vi "Online_Program_redesign_For_TV.vi"() -> ()   [LabVIEW 2014]
uses:
  <vilib>/Utility/file.llb/Read From Spreadsheet File (DBL).vi
  <vilib>/Analysis/Matrix/Numeric/Conversions/Array To Matrix - RA2.vi
  <vilib>/Instr/_visa.llb/VISA Configure Serial Port (Instr).vi
  <vilib>/Analysis/Matrix/Numeric/Conversions/Array To Matrix - RA.vi
  <vilib>/Utility/file.llb/Write To Spreadsheet File (DBL).vi
  <vilib>/Utility/file.llb/Write To Spreadsheet File (I64).vi
  <vilib>/Analysis/Matrix/NI_Matrix.lvlib
  NeuroSky_Dll_Call/Debug/NeuroSky_Dll_Call.dll
  user32.dll
panel:
  out "에러 출력":errorcluster
  out "메시지 2":string
  out "큐사인":bool
  out "icon_온도":bool
  out "icon_용변":bool
  out "icon_자판":bool
  out "icon_응급":bool=TRUE
  out "icon_기계":bool
  out "icon_침대":bool
  out "메시지":string
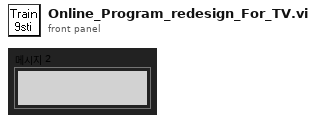
[diagram p1: front panel]
types:
  T1 = typedef "NI_Matrix.lvlib/RealMatrix.ctl" = dbl[][]
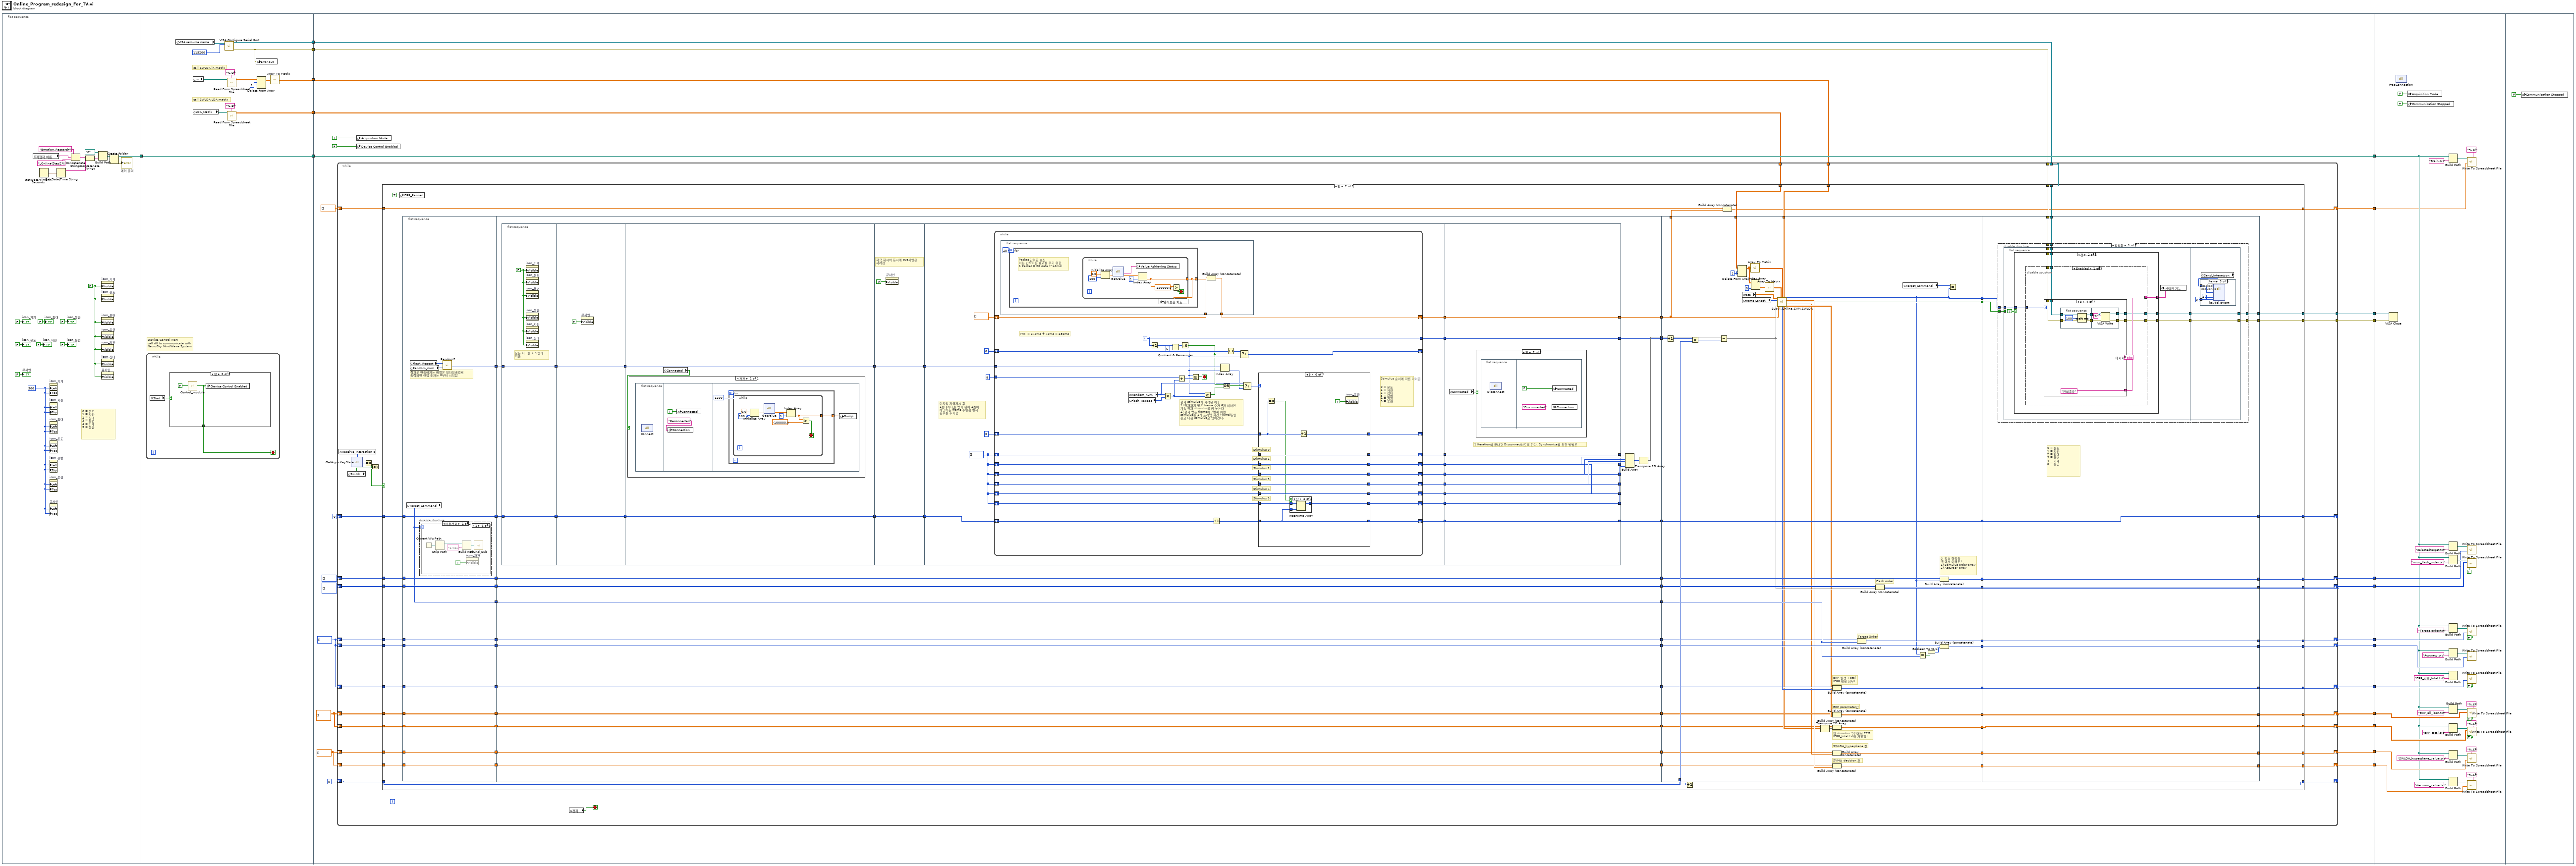
[diagram p0: block diagram]
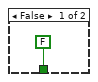
[diagram p2: hidden frame]
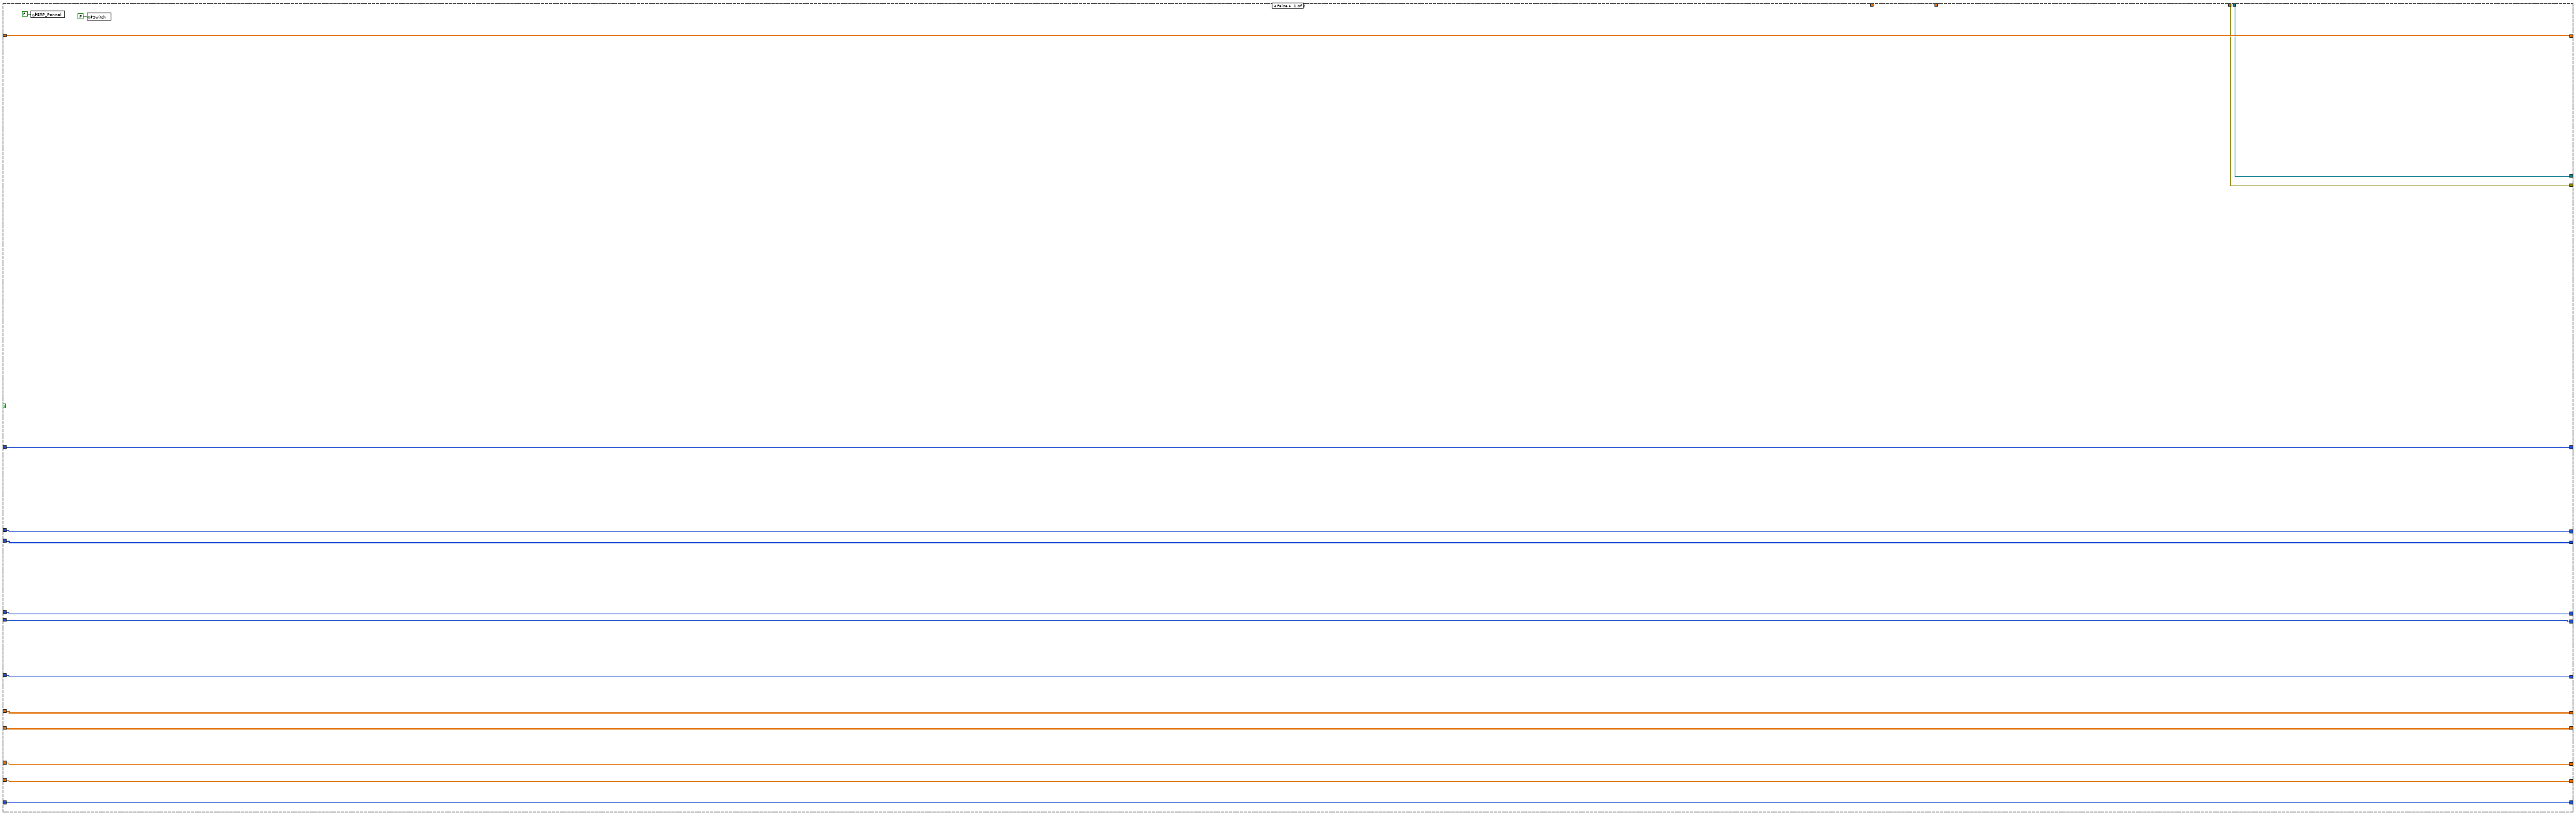
[diagram p3: hidden frame]
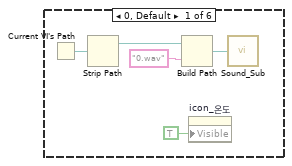
[diagram p4: hidden frame]
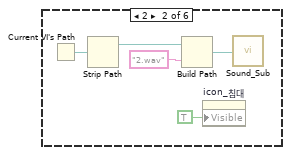
[diagram p5: hidden frame]
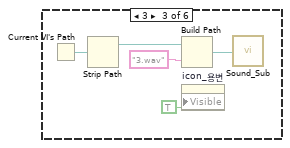
[diagram p6: hidden frame]
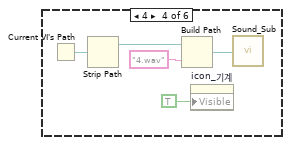
[diagram p7: hidden frame]
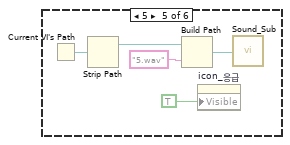
[diagram p8: hidden frame]
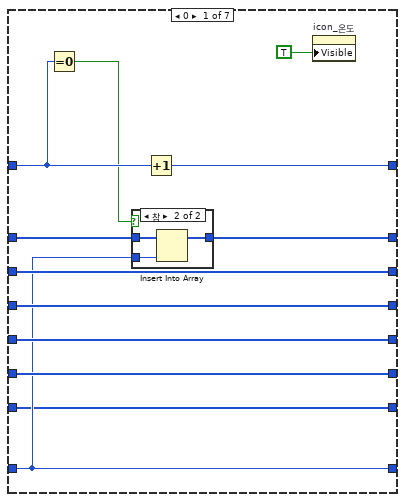
[diagram p11: hidden frame]
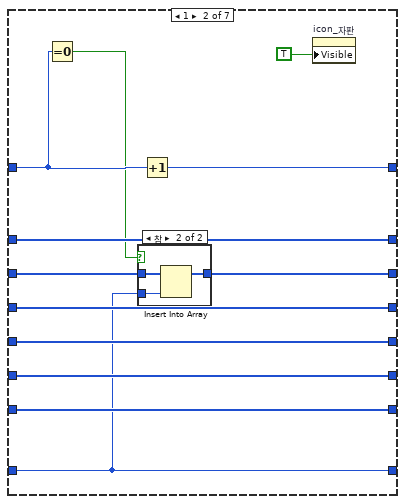
[diagram p13: hidden frame]
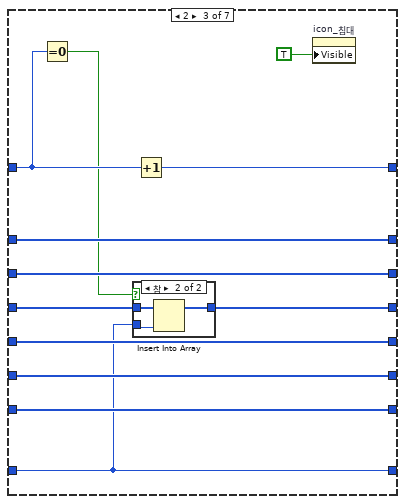
[diagram p15: hidden frame]
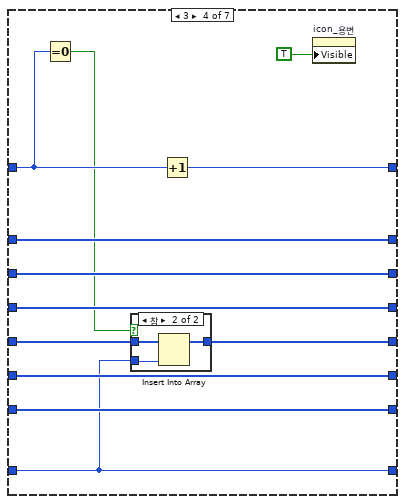
[diagram p17: hidden frame]
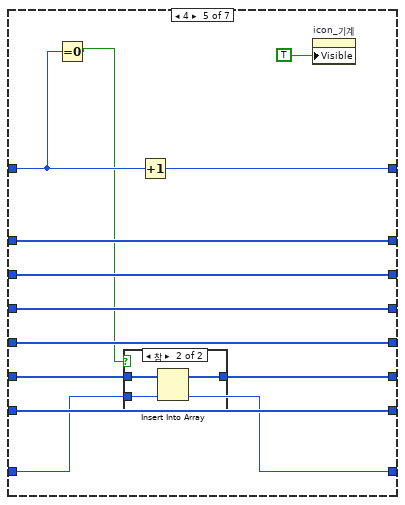
[diagram p19: hidden frame]
diagram:
  n1 = flat-sequence {
    tunnel: [w39] -> w19
    tunnel: w19 -> [w53]
    tunnel: [w53] -> w18
    tunnel: [w51] -> w17
    tunnel: [w44] -> w7
    tunnel: [w43] -> w4
    tunnel: [w40] -> w3
    tunnel: w18 -> [w76]
    tunnel: [w76] -> w16
    tunnel: [w85] -> w15
    tunnel: [w83] -> w14
    tunnel: [w81] -> w13
    tunnel: w17 -> [w65]
    tunnel: [w80] -> w12
    tunnel: [w77] -> w11
    tunnel: [w73] -> w10
    tunnel: [w71] -> w9
    tunnel: [w70] -> w8
    tunnel: w7 -> [w64]
    tunnel: [w68] -> w6
    tunnel: [w66] -> w5
    tunnel: w4 -> [w63]
    tunnel: w3 -> [w62]
    tunnel: [w61] -> w2
    tunnel: [w60] -> w1
    tunnel: w16 -> [w774]
    tunnel: w15 -> [w769]
    tunnel: w14 -> [w808]
    tunnel: w13 -> [w804]
    tunnel: w12 -> [w801]
    tunnel: w11 -> [w797]
    tunnel: w10 -> [w791]
    tunnel: w9 -> [w786]
    tunnel: w8 -> [w783]
    tunnel: w6 -> [w780]
    tunnel: w5 -> [w775]
    tunnel: w2 -> [w771]
    tunnel: w1 -> [w770]
    frame #0 {
      w20 = FALSE ("Visible")
      w22 = 500 ("Position:Left")
      # "0 = 온도\n1 = 자판\n2 = 침대\n3 = 용변 \n4 = 기계 \n5 = 응급"
      n2 = global read "Control_Panel_정리.vi" "피험자 이름"() -> (w30:string)
      n3 = Get Date/Time In Seconds() -> (seconds since 1Jan1904=w36:timestamp)
      n4 = property on="icon_기계" class="Bool (엄격한)"("Left"=w22, "Top"=w22) -> ()  [unwired: 2 in, 2 out]
      n5 = property on="icon_자판" class="Bool (엄격한)"("Left"=w22, "Top"=w22) -> ()  [unwired: 2 in, 2 out]
      n6 = property on="icon_침대" class="Bool (엄격한)"("Left"=w22, "Top"=w22) -> ()  [unwired: 2 in, 2 out]
      n7 = property on="icon_온도" class="Bool (엄격한)"("Left"=w22, "Top"=w22) -> ()  [unwired: 2 in, 2 out]
      n8 = property on="icon_용변" class="Bool (엄격한)"("Left"=w22, "Top"=w22) -> ()  [unwired: 2 in, 2 out]
      n9 = property on="icon_응급" class="Bool (엄격한)"("Left"=w22, "Top"=w22) -> ()  [unwired: 2 in, 2 out]
      n10 = property on="큐사인" class="Bool (엄격한)"("Left"=w22, "Top"=w22) -> ()  [unwired: 2 in, 2 out]
      n11 = Get Date/Time String(seconds (now)=w36) -> (date string=w37:string)  [unwired: 2 in, 1 out]
      n12 = Concatenate Strings("Emotion_Research\\" ("string"), w30, "_Online(Step2)\\" ("문자열")) -> (w32:string)
      n13 = Concatenate Strings(w32, w37) -> (w34:string)
      n14 = Build Path(base path=path "C:/" ("path"), name or relative path=w34) -> (appended path=w35:path)
      n15 = property on="icon_기계" class="Bool (엄격한)"("Visible"=w20) -> ()  [unwired: 2 in, 2 out]
      n16 = property on="icon_온도" class="Bool (엄격한)"("Visible"=w20) -> ()  [unwired: 2 in, 2 out]
      n17 = property on="icon_용변" class="Bool (엄격한)"("Visible"=w20) -> ()  [unwired: 2 in, 2 out]
      n18 = property on="icon_응급" class="Bool (엄격한)"("Visible"=w20) -> ()  [unwired: 2 in, 2 out]
      n19 = property on="icon_자판" class="Bool (엄격한)"("Visible"=w20) -> ()  [unwired: 2 in, 2 out]
      n20 = property on="icon_침대" class="Bool (엄격한)"("Visible"=w20) -> ()  [unwired: 2 in, 2 out]
      n21 = property on="큐사인" class="Bool (엄격한)"("Visible"=w20) -> ()  [unwired: 2 in, 2 out]
      n22 = Create Folder(path (use dialog)=w35) -> (created path=w39:path, error out=→"에러 출력":errorcluster)  [unwired: 2 in, 1 out]
      "icon_온도" <- FALSE ("icon_전원 6")
      "icon_용변" <- FALSE ("icon_전체종료")
      "icon_자판" <- FALSE ("icon_음량업 2")
      "icon_응급" <- FALSE ("icon_채널다운")
      "icon_기계" <- FALSE ("icon_음량다")
      "icon_침대" <- FALSE ("icon_채널업")
      "큐사인" <- FALSE ("icon_전원 7")
    }
    frame #1 {
      w47 = 1 ("인덱스 (행)")
      # "call SWLDA in matrix"
      # "call SWLDA LDA matrix"
      # "Device Control Part\ncall dll to communicate with\nNeuroSky MindWave System"
      n23 = while {
        stop <- w55 stop-if-true
        n24 = global read "Control_Panel_정리.vi" "Start"() -> (w54:bool)
        n25 = case shown="참" w54 {
          tunnel: [FALSE ("Connected") w57] -> w55
          frame False {
          }
          frame True {
            n26 = call "Control_module.vi"("Turn on"=TRUE ("Device Control Enabled")) -> ("Connected"=w57:bool)
            n27 = global write "Control_Panel_정리.vi" "Device Control Enabled"(w57) -> ()
          }
        }
      }
      n28 = global read "Control_Panel_정리.vi" "VISA resource name"() -> (w41:refnum<visa-resource-name>)
      n29 = global read "Control_Panel_정리.vi" "in"() -> (w45:path)
      n30 = global read "Control_Panel_정리.vi" "LDA_Matrix"() -> (w50:path)
      n31 = call-poly "VISA Configure Serial Port"("VISA resource name"=w41, "baud rate (9600)"=u32 115200) -> ("VISA resource name out"=w43:refnum<visa-resource-name>, "error out"=w40:errorcluster)  [unwired: 12 in]
      n32 = call-poly <vilib>:"Read From Spreadsheet File.vi"("format (%.3f)"="%.6f", "file path (dialog if empty)"=w45) -> ("all rows"=w46:dbl[][])  [unwired: 5 in, 4 out]
      n33 = call-poly <vilib>:"Read From Spreadsheet File.vi"("format (%.3f)"="%.6f", "file path (dialog if empty)"=w50) -> ("all rows"=w51:dbl[][])  [unwired: 5 in, 4 out]
      n34 = global write "Control_Panel_정리.vi" "error out"(w40) -> ()
      n35 = Delete From Array(array=w46, length=w47, index (row)=w47) -> (array with subset deleted=w48:dbl[][])  [unwired: 1 in, 1 out]
      n36 = call-poly <vilib>:"Array To Matrix.vi"("Real 2D Array"=w48) -> ("Real Matrix"=w44:T1)
    }
    frame #2 {
      w69 = dbl[] []
      w67 = dbl[][] []
      w72 = i16[] []
      n37 = while {
        shift-right: [w93] -> w85
        shift-left: dbl[] [] -> [w99]
        shift-right: [w119] -> _
        shift-left: 0 ("y") -> [w120]
        shift-right: [w113] -> w83
        shift-left: i32[][] [] -> [w114]
        shift-right: [w117] -> w81
        shift-left: i32[] [] -> [w118]
        shift-right: [w115] -> w80
        shift-left: w72 -> [w116]
        shift-right: [w111] -> w77
        shift-left: w72 -> [w112]
        shift-right: [w110] -> w73
        shift-left: w72 -> [w109]
        shift-right: [w108] -> w71
        shift-left: w67 -> [w107]
        shift-right: [w106] -> w70
        shift-left: w69 -> [w105]
        shift-right: [w104] -> w68
        shift-left: w69 -> [w103]
        shift-right: [w102] -> w66
        shift-left: w67 -> [w101]
        tunnel: w65 -> [w100]
        tunnel: w64 -> [w98]
        tunnel: [w96] -> _
        tunnel: w63 -> [w96]
        tunnel: w62 -> [w97]
        tunnel: [w95] -> w61
        tunnel: [w94] -> w60
        shift-right: [w87] -> _
        shift-left: 0 -> [w88]
        stop <- w89 stop-if-true
        n38 = global read "Control_Panel_정리.vi" "Receive_Interaction"() -> (w91:u8)
        n39 = global read "Control_Panel_정리.vi" "Switch"() -> (w90:bool)
        n40 = dll-call lib="User32.dll" fn="GetAsyncKeyState"("vKey"=w91) -> ("return type"=w92:i64)  [unwired: 4 in, 2 out]
        n41 = Not Equal To 0?(x=w92) -> (x != 0?=w86:bool)
        n42 = Or(x=w86, y=w90) -> ()  [unwired: 1 out]
        n43 = case shown="참" w86 {
          tunnel: w120 -> [w131 w168]
          tunnel: [w131 w167] -> w119
          tunnel: w118 -> [w130 w166]
          tunnel: [w130 w165] -> w117
          tunnel: w116 -> [w127 w164]
          tunnel: [w127 w163] -> w115
          tunnel: w114 -> [w129 w162]
          tunnel: [w129 w161] -> w113
          tunnel: w112 -> [w128 w160]
          tunnel: [w128 w159] -> w111
          tunnel: [w126 w158] -> w110
          tunnel: w109 -> [w126 w157]
          tunnel: [w125 w156] -> w108
          tunnel: w107 -> [w125 w155]
          tunnel: [w123 w154] -> w106
          tunnel: w105 -> [w123 w153]
          tunnel: [w122 w152] -> w104
          tunnel: w103 -> [w122 w151]
          tunnel: [w124 w150] -> w102
          tunnel: w101 -> [w124 w149]
          tunnel: w100 -> [_ w148]
          tunnel: w99 -> [w134 w147]
          tunnel: w98 -> [_ w145]
          tunnel: w97 -> [w132 w144]
          tunnel: w96 -> [w133 w143]
          tunnel: [w133 w142] -> w95
          tunnel: [w132 w141] -> w94
          tunnel: [w134 w140] -> w93
          tunnel: w88 -> [w121 w138]
          tunnel: [w121 w137] -> w87
          frame False {
            n44 = global write "Control_Panel_정리.vi" "ERP_Pannel"(FALSE ("ERP_Pannel")) -> ()
            n45 = global write "Control_Panel_정리.vi" "Switch"(FALSE ("Switch")) -> ()
          }
          frame True {
            n46 = global write "Control_Panel_정리.vi" "ERP_Pannel"(TRUE ("ERP_Pannel")) -> ()
            n47 = flat-sequence {
              tunnel: [w220] -> w206
              tunnel: w168 -> [w219]
              tunnel: [w219] -> w205
              tunnel: [w207] -> w204
              tunnel: w166 -> [w216]
              tunnel: [w216] -> w203
              tunnel: w164 -> [w215]
              tunnel: [w215] -> w202
              tunnel: w162 -> [w214]
              tunnel: [w214] -> w201
              tunnel: [w213] -> w200
              tunnel: w160 -> [w213]
              tunnel: w157 -> [w212]
              tunnel: [w212] -> w199
              tunnel: w155 -> [w211]
              tunnel: [w211] -> w198
              tunnel: w153 -> [w210]
              tunnel: [w210] -> w197
              tunnel: w151 -> [w209]
              tunnel: [w209] -> w196
              tunnel: w149 -> [w208]
              tunnel: [w208] -> w195
              tunnel: w206 -> [w291]
              tunnel: w205 -> [w288]
              tunnel: [w289] -> w194
              tunnel: [w278] -> w193
              tunnel: [w287] -> w192
              tunnel: [w286] -> w191
              tunnel: w204 -> [w285]
              tunnel: [w285] -> w190
              tunnel: w203 -> [w284]
              tunnel: [w284] -> w189
              tunnel: [w283] -> w188
              tunnel: w202 -> [w283]
              tunnel: [w282] -> w187
              tunnel: w201 -> [w282]
              tunnel: [w281] -> w186
              tunnel: w200 -> [w281]
              tunnel: [w280] -> w185
              tunnel: w199 -> [w280]
              tunnel: [w279] -> w184
              tunnel: w198 -> [w279]
              tunnel: [w277] -> w183
              tunnel: w197 -> [w277]
              tunnel: [w276] -> w182
              tunnel: w196 -> [w276]
              tunnel: w195 -> [w275]
              tunnel: [w275] -> w181
              tunnel: w194 -> [w532]
              tunnel: w193 -> [w506]
              tunnel: w192 -> [w545]
              tunnel: w191 -> [w546]
              tunnel: w138 -> [w544]
              tunnel: [w545] -> w170
              tunnel: [w504] -> w171
              tunnel: w190 -> [w531]
              tunnel: w189 -> [w540]
              tunnel: [w539] -> w172
              tunnel: w188 -> [w537]
              tunnel: [w536] -> w173
              tunnel: w187 -> [w535]
              tunnel: [w533] -> w174
              tunnel: w186 -> [w530]
              tunnel: [w529] -> w175
              tunnel: [w527] -> w176
              tunnel: w185 -> [w526]
              tunnel: [w524] -> w177
              tunnel: w184 -> [w523]
              tunnel: [w521] -> w178
              tunnel: w183 -> [w520]
              tunnel: [w518] -> w179
              tunnel: w182 -> [w517]
              tunnel: [w514] -> w180
              tunnel: w181 -> [w513]
              tunnel: w148 -> [w512]
              tunnel: [w506] -> w146
              tunnel: w145 -> [w508]
              tunnel: [w507] -> w169
              tunnel: [w567] -> w167
              tunnel: [w566] -> w165
              tunnel: [w563] -> w163
              tunnel: [w565] -> w161
              tunnel: [w564] -> w159
              tunnel: [w562] -> w158
              tunnel: [w561] -> w156
              tunnel: [w560] -> w154
              tunnel: [w559] -> w152
              tunnel: [w558] -> w150
              tunnel: w180 -> [w558]
              tunnel: w179 -> [w559]
              tunnel: w178 -> [w560]
              tunnel: w177 -> [w561]
              tunnel: w176 -> [w562]
              tunnel: w175 -> [w564]
              tunnel: w174 -> [w565]
              tunnel: w173 -> [w563]
              tunnel: w172 -> [w566]
              tunnel: w171 -> [w557]
              tunnel: w170 -> [w567]
              tunnel: w169 -> [w556]
              tunnel: w144 -> [w555]
              tunnel: w143 -> [w554]
              tunnel: [w553] -> w142
              tunnel: [w552] -> w141
              frame #0 {
                # "결과로 만들어지는 배열은 일차원배열로\n출력되면 랜덤 숫자는 0부터 시작함"
                n48 = global read "Control_Panel_정리.vi" "Target_Command"() -> (w207:i32)
                n49 = global read "Control_Panel_정리.vi" "Flash_Repeat"() -> (w218:i32)
                n50 = global read "Control_Panel_정리.vi" "Random_num"() -> (w217:i32)
                n51 = disable-structure shown="비활성화" {
                  disable-tunnel: w207 -> [w221 _]
                  frame Disabled {
                    n52 = case shown="1" w221 {
                      frame 0, Default {
                        n53 = Current VI's Path() -> (path=w224:path)
                        n54 = Strip Path(path=w224) -> (stripped path=w225:path)  [unwired: 1 out]
                        n55 = Build Path(base path=w225, name or relative path="0.wav" ("이름 또는 상대 경로")) -> (appended path=w223:path)
                        n56 = property on="icon_온도" class="Bool (엄격한)"("Visible"=TRUE) -> ()  [unwired: 2 in, 2 out]
                        n57 = call "Sound_Sub.vi"("path"=w223) -> ()
                      }
                      frame 2 {
                        n58 = Current VI's Path() -> (path=w228:path)
                        n59 = Strip Path(path=w228) -> (stripped path=w229:path)  [unwired: 1 out]
                        n60 = Build Path(base path=w229, name or relative path="2.wav" ("이름 또는 상대 경로")) -> (appended path=w231:path)
                        n61 = property on="icon_침대" class="Bool (엄격한)"("Visible"=TRUE) -> ()  [unwired: 2 in, 2 out]
                        n62 = call "Sound_Sub.vi"("path"=w231) -> ()
                      }
                      frame 3 {
                        n63 = Current VI's Path() -> (path=w233:path)
                        n64 = Strip Path(path=w233) -> (stripped path=w234:path)  [unwired: 1 out]
                        n65 = Build Path(base path=w234, name or relative path="3.wav" ("이름 또는 상대 경로")) -> (appended path=w236:path)
                        n66 = property on="icon_용변" class="Bool (엄격한)"("Visible"=TRUE) -> ()  [unwired: 2 in, 2 out]
                        n67 = call "Sound_Sub.vi"("path"=w236) -> ()
                      }
                      frame 4 {
                        n68 = Current VI's Path() -> (path=w238:path)
                        n69 = Strip Path(path=w238) -> (stripped path=w239:path)  [unwired: 1 out]
                        n70 = Build Path(base path=w239, name or relative path="4.wav" ("이름 또는 상대 경로")) -> (appended path=w241:path)
                        n71 = property on="icon_기계" class="Bool (엄격한)"("Visible"=TRUE) -> ()  [unwired: 2 in, 2 out]
                        n72 = call "Sound_Sub.vi"("path"=w241) -> ()
                      }
                      frame 5 {
                        n73 = Current VI's Path() -> (path=w243:path)
                        n74 = Strip Path(path=w243) -> (stripped path=w244:path)  [unwired: 1 out]
                        n75 = Build Path(base path=w244, name or relative path="5.wav" ("이름 또는 상대 경로")) -> (appended path=w246:path)
                        n76 = property on="icon_응급" class="Bool (엄격한)"("Visible"=TRUE) -> ()  [unwired: 2 in, 2 out]
                        n77 = call "Sound_Sub.vi"("path"=w246) -> ()
                      }
                      frame 1 {
                        n78 = Current VI's Path() -> (path=w249:path)
                        n79 = Strip Path(path=w249) -> (stripped path=w250:path)  [unwired: 1 out]
                        n80 = Build Path(base path=w250, name or relative path="1.wav" ("이름 또는 상대 경로")) -> (appended path=w248:path)
                        n81 = property on="icon_자판" class="Bool (엄격한)"("Visible"=TRUE) -> ()  [unwired: 2 in, 2 out]
                        n82 = call "Sound_Sub.vi"("path"=w248) -> ()
                      }
                    }
                  }
                  frame Enabled {
                  }
                }
                n83 = call "Random2.vi"("Random_num"=w217, "전체횟수"=w218) -> ("배열"=w220:i32[])
              }
              frame #1 {
                n84 = flat-sequence {
                  tunnel: w288 -> [w293]
                  tunnel: w291 -> [w294]
                  tunnel: [w294] -> w274
                  tunnel: [w293] -> w273
                  tunnel: [w297] -> w266
                  tunnel: [w296] -> w265
                  tunnel: w274 -> [w297]
                  tunnel: w273 -> [w296]
                  tunnel: w266 -> [w300]
                  tunnel: [w300] -> w255
                  tunnel: w265 -> [w299]
                  tunnel: [w299] -> w253
                  tunnel: w255 -> [w316]
                  tunnel: [w316] -> w254
                  tunnel: w253 -> [w315]
                  tunnel: [w315] -> w252
                  tunnel: w254 -> [w332]
                  tunnel: w252 -> [w322]
                  tunnel: [w330] -> w264
                  tunnel: [w329] -> w263
                  tunnel: [w328] -> w262
                  tunnel: [w327] -> w261
                  tunnel: [w326] -> w260
                  tunnel: [w321] -> w259
                  tunnel: [w320] -> w258
                  tunnel: [w319] -> w257
                  tunnel: [w317] -> w256
                  tunnel: [w493] -> w278
                  tunnel: [w494] -> w269
                  tunnel: [w495] -> w286
                  tunnel: [w496] -> w287
                  tunnel: [w497] -> w272
                  tunnel: [w498] -> w271
                  tunnel: [w499] -> w270
                  tunnel: [w500] -> w268
                  tunnel: [w501] -> w267
                  tunnel: w264 -> [w501]
                  tunnel: w263 -> [w500]
                  tunnel: w262 -> [w499]
                  tunnel: w261 -> [w498]
                  tunnel: w260 -> [w497]
                  tunnel: w259 -> [w496]
                  tunnel: w258 -> [w495]
                  tunnel: w257 -> [w494]
                  tunnel: w256 -> [w493]
                  frame #0 {
                    w292 = FALSE ("Visible")
                    # "모든 자극을 시작전에\n꺼줌"
                    n85 = property on="icon_기계" class="Bool (엄격한)"("Visible"=w292) -> ()  [unwired: 2 in, 2 out]
                    n86 = property on="icon_온도" class="Bool (엄격한)"("Visible"=w292) -> ()  [unwired: 2 in, 2 out]
                    n87 = property on="icon_용변" class="Bool (엄격한)"("Visible"=w292) -> ()  [unwired: 2 in, 2 out]
                    n88 = property on="icon_응급" class="Bool (엄격한)"("Visible"=w292) -> ()  [unwired: 2 in, 2 out]
                    n89 = property on="icon_자판" class="Bool (엄격한)"("Visible"=w292) -> ()  [unwired: 2 in, 2 out]
                    n90 = property on="icon_침대" class="Bool (엄격한)"("Visible"=w292) -> ()  [unwired: 2 in, 2 out]
                  }
                  frame #1 {
                    n91 = property on="큐사인" class="Bool (엄격한)"("Visible"=TRUE) -> ()  [unwired: 2 in, 2 out]
                  }
                  frame #2 {
                    n92 = global read "Control_Panel_정리.vi" "Connected"() -> (w298:bool)
                    n93 = case shown="거짓" w298 {
                      frame False {
                        n94 = flat-sequence {
                          frame #0 {
                            n95 = dll-call lib="C:/Users/Server/Desktop/NeuroSky/NeuroSky_Dll_Call/Debug/NeuroSky_Dll_Call.dll" fn="Connect"() -> ()  [unwired: 4 in, 2 out]
                          }
                          frame #1 {
                            n96 = global write "Control_Panel_정리.vi" "Connection"("Reconnected") -> ()
                            n97 = global write "Control_Panel_정리.vi" "Connected"(TRUE ("Connected")) -> ()
                          }
                          frame #2 {
                            n98 = for {
                              N: 1200 -> [_]
                              tunnel: [w305] -> w303 mode=indexing
                              n99 = while {
                                tunnel: [w307] -> w305
                                stop <- w306 stop-if-true
                                n100 = Initialize Array(0.0 ("element"), 100 ("dimension size")) -> (w312:dbl[])
                                n101 = dll-call lib="C:/Users/Server/Desktop/NeuroSky/NeuroSky_Dll_Call/Debug/NeuroSky_Dll_Call.dll" fn="GetValue"("result"=w312) -> ("result"=w313:dbl[])  [unwired: 4 in, 2 out]
                                n102 = Index Array(array=w313, index=1) -> (element=w307:dbl)
                                n103 = Greater?(x=w307, y=-100000.0) -> (0:w306:bool)
                              }
                            }
                            n104 = global write "Control_Panel_정리.vi" "Dump"(w303) -> ()
                          }
                        }
                      }
                      frame True {
                      }
                    }
                  }
                  frame #3 {
                    # "자극 제시와 동시에 cue사인은\n사라짐"
                    n105 = property on="큐사인" class="Bool (엄격한)"("Visible"=FALSE) -> ()  [unwired: 2 in, 2 out]
                  }
                  frame #4 {
                    w324 = i32[] []
                    # "마지막 자극제시 후\n1초데이터를 받기 위해 2초에\n해당하는 frame 수만큼 반복\n횟수를 추가함"
                    n106 = while {
                      tunnel: w332 -> [w368]
                      shift-right: [w336] -> w317
                      shift-left: dbl[] [] -> [w337]
                      tunnel: 8 -> [w333]
                      shift-right: [w365] -> w330
                      shift-left: w324 -> [w364]
                      shift-right: [w362] -> w329
                      shift-left: w324 -> [w363]
                      shift-right: [w360] -> w319
                      shift-left: w324 -> [w361]
                      shift-right: [w358] -> w328
                      shift-left: w324 -> [w359]
                      shift-right: [w356] -> w327
                      shift-left: w324 -> [w357]
                      shift-right: [w355] -> w326
                      shift-left: w324 -> [w342]
                      shift-right: [w353] -> w321
                      shift-left: w322 -> [w354]
                      shift-right: [w349] -> _
                      shift-left: 0 -> [w348]
                      shift-right: [w343] -> _
                      shift-left: 0 ("y") -> [w344]
                      tunnel: [w338] -> w320
                      i -> [w338]
                      stop <- w369 stop-if-true
                      # "ITR  = 240ms + 40ms = 280ms"
                      # "현재 stimulus가 시작된 이후\n1) 현재까지 받은 frame 수가 6개 이하면\n계속 현재 stimulus를 켜 놓는다\n2) 현재 받는 frame이 7번째 이면\nstimulus를 1개 프레임 시간 (40ms)동안\n끈고 다음 stimulus로 넘어간다."
                      # "Stimulus 순서에 따른 아이콘\n\n\n0 = 온도\n1 = 자판\n2 = 침대\n3 = 용변 \n4 = 기계 \n5 = 응급"
                      # "Stimulus 5"
                      # "Stimulus 4"
                      # "Stimulus 3"
                      # "Stimulus 2"
                      # "Stimulus 1"
                      # "Stimulus 0"
                      n107 = flat-sequence {
                        tunnel: [w374] -> w336
                        tunnel: w337 -> [w373]
                        frame #0 {
                          n108 = for {
                            N: 20 -> [_]
                            tunnel: [w375] -> w372 mode=indexing
                            # "Packet 단위로 송신\n이는 반짝이는 효과를 주기 위함\n1 Packet = 20 data (~40ms)"
                            n109 = while {
                              tunnel: [w377] -> w375
                              stop <- w376 stop-if-true
                              n110 = Initialize Array(0.0 ("element"), 100 ("dimension size")) -> (w383:dbl[])
                              n111 = dll-call lib="C:/Users/Server/Desktop/NeuroSky/NeuroSky_Dll_Call/Debug/NeuroSky_Dll_Call.dll" fn="GetValue"("result"=w383) -> ("errCode"=w379:string, "result"=w384:dbl[])  [unwired: 3 in, 2 out]
                              n112 = global write "Control_Panel_정리.vi" "Value Achieving Status"(w379) -> ()
                              n113 = Index Array(array=w384, index=1) -> (element=w377:dbl)
                              n114 = Greater?(x=w377, y=-100000.0) -> (0:w376:bool)
                            }
                            n115 = global write "Control_Panel_정리.vi" "웨이브폼 차트"(w375) -> ()
                          }
                          n116 = Build Array (concatenate)(w373, w372) -> (w374:dbl[])
                        }
                      }
                      n117 = global read "Control_Panel_정리.vi" "Random_num"() -> (w335:i32)
                      n118 = global read "Control_Panel_정리.vi" "Flash_Repeat"() -> (w334:i32)
                      n119 = Increment(x=w338) -> (x+1=w341:i32)
                      n120 = Multiply(x=w335, y=w334) -> (x*y=w339:i32)
                      n121 = Quotient & Remainder(x=w341, y=6) -> (x-y*floor(x/y)=w351:i32)  [unwired: 1 out]
                      n122 = Add(x=w333, y=w339) -> (x+y=w370:i32)
                      n123 = Equal To 0?(x=w351) -> (x = 0?=w347:bool)
                      n124 = Greater Or Equal?(x=w348, y=w370) -> (x >= y?=w369:bool)
                      n125 = Greater Or Equal?(x=w348, y=w339) -> (x >= y?=w346:bool)
                      n126 = Increment(x=w354) -> (x+1=w366:i32)
                      n127 = Index Array(array=w368, index=w348) -> (element=w340:i32)
                      n128 = Or(x=w347, y=w346) -> (x .or. y?=w345:bool)
                      n129 = Increment(x=w348) -> (x+1=w350:i32)
                      n130 = Select(t=w350, s=w347, f=w348) -> (s? t:f=w349:i32)
                      n131 = Select(t=w335, s=w345, f=w340) -> (s? t:f=w367:i32)
                      n132 = case shown="5" w367 {
                        tunnel: w366 -> [w390 w406 w421 w437 w453 w470 w485]
                        tunnel: [w395 w403 w428 w444 w460 w476 w491] -> w365
                        tunnel: w364 -> [w396 w403 w428 w444 w460 w476 w491]
                        tunnel: w363 -> [w394 w412 w425 w441 w457 w474 w490]
                        tunnel: [w394 w411 w425 w441 w457 w474 w490] -> w362
                        tunnel: w361 -> [w393 w410 w427 w440 w456 w473 w489]
                        tunnel: [w393 w410 w426 w440 w456 w473 w489] -> w360
                        tunnel: w359 -> [w392 w409 w424 w443 w455 w472 w488]
                        tunnel: [w392 w409 w424 w442 w455 w472 w488] -> w358
                        tunnel: w357 -> [w391 w408 w423 w439 w459 w471 w487]
                        tunnel: [w391 w408 w423 w439 w458 w471 w487] -> w356
                        tunnel: w342 -> [w387 w407 w422 w438 w454 w475 w486]
                        tunnel: [w387 w407 w422 w438 w454 w467 w486] -> w355
                        tunnel: [w390 w406 w421 w437 w453 w470 w485] -> w353
                        tunnel: w344 -> [w389 w405 w420 w435 w452 w468 _]
                        tunnel: [w388 w404 w419 w436 w451 w469 0] -> w343
                        frame 0 {
                          n133 = Equal To 0?(x=w389) -> (x = 0?=w385:bool)
                          n134 = case shown="참" w385 {
                            tunnel: w396 -> [w397 w400]
                            tunnel: [w397 w399] -> w395
                            tunnel: w390 -> [_ w398]
                            frame False {
                            }
                            frame True {
                              n135 = Insert Into Array(array=w400, new element=w398) -> (w399:i32[])  [unwired: 1 in]
                            }
                          }
                          n136 = Increment(x=w389) -> (x+1=w388:i32)
                          n137 = property on="icon_온도" class="Bool (엄격한)"("Visible"=TRUE) -> ()  [unwired: 2 in, 2 out]
                        }
                        frame 1 {
                          n138 = Equal To 0?(x=w405) -> (x = 0?=w401:bool)
                          n139 = case shown="참" w401 {
                            tunnel: w412 -> [w413 w416]
                            tunnel: [w413 w415] -> w411
                            tunnel: w406 -> [_ w414]
                            frame False {
                            }
                            frame True {
                              n140 = Insert Into Array(array=w416, new element=w414) -> (w415:i32[])  [unwired: 1 in]
                            }
                          }
                          n141 = Increment(x=w405) -> (x+1=w404:i32)
                          n142 = property on="icon_자판" class="Bool (엄격한)"("Visible"=TRUE) -> ()  [unwired: 2 in, 2 out]
                        }
                        frame 2 {
                          n143 = Equal To 0?(x=w420) -> (x = 0?=w417:bool)
                          n144 = case shown="참" w417 {
                            tunnel: w427 -> [w429 w432]
                            tunnel: [w429 w431] -> w426
                            tunnel: w421 -> [_ w430]
                            frame False {
                            }
                            frame True {
                              n145 = Insert Into Array(array=w432, new element=w430) -> (w431:i32[])  [unwired: 1 in]
                            }
                          }
                          n146 = Increment(x=w420) -> (x+1=w419:i32)
                          n147 = property on="icon_침대" class="Bool (엄격한)"("Visible"=TRUE) -> ()  [unwired: 2 in, 2 out]
                        }
                        frame 3 {
                          n148 = Equal To 0?(x=w435) -> (x = 0?=w433:bool)
                          n149 = case shown="참" w433 {
                            tunnel: w443 -> [w445 w448]
                            tunnel: [w445 w447] -> w442
                            tunnel: w437 -> [_ w446]
                            frame False {
                            }
                            frame True {
                              n150 = Insert Into Array(array=w448, new element=w446) -> (w447:i32[])  [unwired: 1 in]
                            }
                          }
                          n151 = Increment(x=w435) -> (x+1=w436:i32)
                          n152 = property on="icon_용변" class="Bool (엄격한)"("Visible"=TRUE) -> ()  [unwired: 2 in, 2 out]
                        }
                        frame 4 {
                          n153 = Equal To 0?(x=w452) -> (x = 0?=w449:bool)
                          n154 = case shown="참" w449 {
                            tunnel: w459 -> [w461 w464]
                            tunnel: [w461 w463] -> w458
                            tunnel: w453 -> [_ w462]
                            frame False {
                            }
                            frame True {
                              n155 = Insert Into Array(array=w464, new element=w462) -> (w463:i32[])  [unwired: 1 in]
                            }
                          }
                          n156 = Increment(x=w452) -> (x+1=w451:i32)
                          n157 = property on="icon_기계" class="Bool (엄격한)"("Visible"=TRUE) -> ()  [unwired: 2 in, 2 out]
                        }
                        frame 5 {
                          n158 = Equal To 0?(x=w468) -> (x = 0?=w465:bool)
                          n159 = case shown="참" w465 {
                            tunnel: w475 -> [w477 w480]
                            tunnel: [w477 w479] -> w467
                            tunnel: w470 -> [_ w478]
                            frame False {
                            }
                            frame True {
                              n160 = Insert Into Array(array=w480, new element=w478) -> (w479:i32[])  [unwired: 1 in]
                            }
                          }
                          n161 = Increment(x=w468) -> (x+1=w469:i32)
                          n162 = property on="icon_응급" class="Bool (엄격한)"("Visible"=TRUE) -> ()  [unwired: 2 in, 2 out]
                        }
                        frame 6, Default {
                          w482 = FALSE ("Visible")
                          w483 = FALSE ("Visible")
                          w481 = FALSE ("Visible")
                          n163 = property on="icon_기계" class="Bool (엄격한)"("Visible"=w481) -> ()  [unwired: 2 in, 2 out]
                          n164 = property on="icon_온도" class="Bool (엄격한)"("Visible"=w481) -> ()  [unwired: 2 in, 2 out]
                          n165 = property on="icon_응급" class="Bool (엄격한)"("Visible"=w483) -> ()  [unwired: 2 in, 2 out]
                          n166 = property on="icon_용변" class="Bool (엄격한)"("Visible"=w483) -> ()  [unwired: 2 in, 2 out]
                          n167 = property on="icon_자판" class="Bool (엄격한)"("Visible"=w482) -> ()  [unwired: 2 in, 2 out]
                          n168 = property on="icon_침대" class="Bool (엄격한)"("Visible"=w482) -> ()  [unwired: 2 in, 2 out]
                        }
                      }
                    }
                  }
                  frame #5 {
                    # "1 Iteration이 끝나고 Disconnect하도록 한다. Synchronize를 위한 방법론"
                    n169 = global read "Control_Panel_정리.vi" "Connected"() -> (w492:bool)
                    n170 = case shown="참" w492 {
                      frame False {
                      }
                      frame True {
                        n171 = flat-sequence {
                          frame #0 {
                            n172 = dll-call lib="C:/Users/Server/Desktop/NeuroSky/NeuroSky_Dll_Call/Debug/NeuroSky_Dll_Call.dll" fn="Disconnect"() -> ()  [unwired: 4 in, 2 out]
                          }
                          frame #1 {
                            n173 = global write "Control_Panel_정리.vi" "Connection"("Disconnected") -> ()
                            n174 = global write "Control_Panel_정리.vi" "Connected"(FALSE ("Connected")) -> ()
                          }
                        }
                      }
                    }
                  }
                }
                n175 = Build Array(w267, w268, w269, w270, w271, w272) -> (w290:i32[][])
                n176 = Transpose 2D Array(2D array=w290) -> (transposed array=w289:i32[][])
              }
              frame #2 {
                w549 = 1 ("인덱스 (행)")
                # "각 stimulus 구간에서 EEG\n(ERP_total.txt라 저장됨)"
                # "ERP parameter값"
                # "SVM의 decision 값"
                # "SWLDA_hyperplane 값"
                # "ERP_발생_Total\n(ERP 발생 여부)"
                # "Target Order"
                # "Flash order"
                # "이 열의 행렬들 \n(위에서 아래로)\n1) Stimulus order array\n2) Accuracy array"
                n177 = Increment(x=w546) -> (x+1=w550:i32)
                n178 = Multiply(x=w550, y=w544) -> (x*y=w551:i32)
                n179 = Subtract(x=w532, y=w551) -> (x-y=w534:i32[][])
                n180 = Delete From Array(array=w512, length=w549, index (row)=w549) -> (array with subset deleted=w510:dbl[][])  [unwired: 1 in, 1 out]
                n181 = global read "Control_Panel_정리.vi" "rate"() -> (w542:dbl)
                n182 = global read "Control_Panel_정리.vi" "Frame Length"() -> (w543:i32)
                n183 = call-poly <vilib>:"Array To Matrix.vi"("Real 2D Array"=w510) -> ("Real Matrix"=w509:T1)
                n184 = Index Array(array=w510, index (col)=0 ("인덱스")) -> (element=w511:dbl[])  [unwired: 1 in]
                n185 = call-poly <vilib>:"Array To Matrix.vi"("Real 1D Array"=w511) -> ("Real Matrix (Column Vector)"=w547:T1)
                n186 = call "Subvi_Online_SVM_SWLDA.vi"("rate"=w542, "Value"=w547, "Matrix"=w509, "in"=w508, "samples per channel"=w543, "Brain_data_source"=w506, "Target_Flash_Order"=w534) -> ("output-0~8"=w504:i32, "decision"=w519:dbl[], "ERP_발생여부"=w507:bool, "SWLDA"=w522:dbl[], "EPR_발생_total"=w528:i16[], "ERP_all"=w516:dbl[][], "ERP_Parameters"=w525:dbl[][])  [unwired: 2 in]
                n187 = Transpose 2D Array(2D array=w516) -> (transposed array=w515:dbl[][])
                n188 = Build Array (concatenate)(w526, w528) -> (w527:i16[])
                n189 = Build Array (concatenate)(w523, w525) -> (w524:dbl[][])
                n190 = Build Array (concatenate)(w513, w515) -> (w514:dbl[][])
                n191 = Build Array (concatenate)(w520, w522) -> (w521:dbl[])
                n192 = Build Array (concatenate)(w517, w519) -> (w518:dbl[])
                n193 = Build Array (concatenate)(w530, w531) -> (w529:i32[])
                n194 = Build Array (concatenate)(w535, w534) -> (w533:i32[][])
                n195 = global read "Control_Panel_정리.vi" "Target_Command"() -> (w505:i32)
                n196 = Equal?(x=w504, y=w531) -> (x = y?=w541:bool)
                n197 = Boolean To (0,1)(Boolean=w541) -> (0, 1=w538:i16)
                n198 = Build Array (concatenate)(w540, w504) -> (w539:i32[])
                n199 = Build Array (concatenate)(w537, w538) -> (w536:i16[])
                n200 = Equal?(x=w505, y=w504) -> ()  [unwired: 1 out]
              }
              frame #3 {
                # "0 = 온도\n1 = 자판\n2 = 침대\n3 = 용변 \n4 = 기계 \n5 = 응급"
                n201 = disable-structure shown="활성화" {
                  disable-tunnel: w557 -> [w575 w730]
                  disable-tunnel: w556 -> [w574 w729]
                  disable-tunnel: w555 -> [w573 _]
                  disable-tunnel: w554 -> [w572 _]
                  disable-tunnel: [w571 _] -> w553
                  disable-tunnel: [w570 _] -> w552
                  frame Enabled {
                    n202 = flat-sequence {
                      tunnel: w575 -> [w582]
                      tunnel: w574 -> [_]
                      tunnel: w573 -> [w581]
                      tunnel: w572 -> [w580]
                      tunnel: [w579] -> w569
                      tunnel: [w578] -> w568
                      tunnel: [w719] -> w570
                      tunnel: [w720] -> w571
                      tunnel: w569 -> [w720]
                      tunnel: w568 -> [w719]
                      frame #0 {
                        n203 = case shown="참" TRUE {
                          tunnel: w582 -> [_ w591]
                          tunnel: ["No Decesion" ("메시지") w590] -> w577
                          tunnel: w581 -> [w583 w589]
                          tunnel: w580 -> [w584 w588]
                          tunnel: [w584 w587] -> w579
                          tunnel: [w583 w586] -> w578
                          frame False {
                          }
                          frame True {
                            n204 = disable-structure shown="Enabled" {
                              disable-tunnel: [w597 _ "" ("메시지")] -> w590
                              disable-tunnel: w591 -> [w592 w691 _]
                              disable-tunnel: w589 -> [w596 _ _]
                              disable-tunnel: w588 -> [w595 _ _]
                              disable-tunnel: [w594 _ _] -> w587
                              disable-tunnel: [w593 _ _] -> w586
                              frame Enabled {
                                n205 = case shown="3" w592 {
                                tunnel: ["전원" ("메시지") "음향 UP" ("메시지") "채널 UP" ("메시지") "전체종료" ("메시지") "음향 Down" ("메시지") "채널 Down" ("메시지") "No Decesion" ("메시지")] -> w597
                                tunnel: w596 -> [w603 w618 w633 w645 w663 w678 w688]
                                tunnel: w595 -> [w599 w614 w629 w646 w659 w674 w689]
                                tunnel: [w602 w617 w632 w644 w662 w677 w689] -> w594
                                tunnel: [w601 w616 w631 w643 w661 w676 w688] -> w593
                                frame 0 {
                                n206 = flat-sequence {
                                tunnel: w603 -> [w607]
                                tunnel: [w607] -> w600
                                tunnel: w599 -> [w606]
                                tunnel: [w606] -> w598
                                tunnel: [w610] -> w602
                                tunnel: [w609] -> w601
                                tunnel: w600 -> [w611]
                                tunnel: w598 -> [w608]
                                frame #0 {
                                n207 = Wait (ms)(milliseconds to wait=u32 100) -> ()  [unwired: 1 out]
                                }
                                frame #1 {
                                n208 = VISA Write(VISA resource name=w608, write buffer="0", error in (no error)=w611) -> (VISA resource name out=w610:refnum<visa-resource-name>, error out=w609:errorcluster)  [unwired: 1 out]
                                }
                                }
                                }
                                frame 1 {
                                n209 = flat-sequence {
                                tunnel: w618 -> [w622]
                                tunnel: [w622] -> w615
                                tunnel: w614 -> [w621]
                                tunnel: [w621] -> w613
                                tunnel: [w625] -> w617
                                tunnel: [w624] -> w616
                                tunnel: w615 -> [w626]
                                tunnel: w613 -> [w623]
                                frame #0 {
                                n210 = Wait (ms)(milliseconds to wait=u32 100) -> ()  [unwired: 1 out]
                                }
                                frame #1 {
                                n211 = VISA Write(VISA resource name=w623, write buffer="L", error in (no error)=w626) -> (VISA resource name out=w625:refnum<visa-resource-name>, error out=w624:errorcluster)  [unwired: 1 out]
                                }
                                }
                                }
                                frame 2 {
                                n212 = flat-sequence {
                                tunnel: w633 -> [w637]
                                tunnel: [w637] -> w630
                                tunnel: [w636] -> _
                                tunnel: w629 -> [w636]
                                tunnel: [w636] -> w628
                                tunnel: [w640] -> w632
                                tunnel: [w639] -> w631
                                tunnel: w630 -> [w641]
                                tunnel: w628 -> [w638]
                                frame #0 {
                                n213 = Wait (ms)(milliseconds to wait=u32 100) -> ()  [unwired: 1 out]
                                }
                                frame #1 {
                                n214 = VISA Write(VISA resource name=w638, write buffer="J", error in (no error)=w641) -> (VISA resource name out=w640:refnum<visa-resource-name>, error out=w639:errorcluster)  [unwired: 1 out]
                                }
                                }
                                }
                                frame 3 {
                                n215 = flat-sequence {
                                tunnel: w645 -> [w652]
                                tunnel: [w652] -> w648
                                tunnel: w646 -> [w651]
                                tunnel: [w651] -> w647
                                tunnel: [w655] -> w644
                                tunnel: [w654] -> w643
                                tunnel: w648 -> [w656]
                                tunnel: w647 -> [w653]
                                frame #0 {
                                n216 = Wait (ms)(milliseconds to wait=u32 100) -> ()  [unwired: 1 out]
                                }
                                frame #1 {
                                n217 = VISA Write(VISA resource name=w653, write buffer="0", error in (no error)=w656) -> (VISA resource name out=w655:refnum<visa-resource-name>, error out=w654:errorcluster)  [unwired: 1 out]
                                }
                                }
                                }
                                frame 4 {
                                n218 = flat-sequence {
                                tunnel: w663 -> [w667]
                                tunnel: [w667] -> w660
                                tunnel: w659 -> [w665]
                                tunnel: [w665] -> w658
                                tunnel: [w670] -> w662
                                tunnel: [w669] -> w661
                                tunnel: w660 -> [w671]
                                tunnel: w658 -> [w668]
                                frame #0 {
                                n219 = Wait (ms)(milliseconds to wait=u32 100) -> ()  [unwired: 1 out]
                                }
                                frame #1 {
                                n220 = VISA Write(VISA resource name=w668, write buffer="M", error in (no error)=w671) -> (VISA resource name out=w670:refnum<visa-resource-name>, error out=w669:errorcluster)  [unwired: 1 out]
                                }
                                }
                                }
                                frame 5 {
                                n221 = flat-sequence {
                                tunnel: w678 -> [w682]
                                tunnel: [w682] -> w675
                                tunnel: w674 -> [w681]
                                tunnel: [w681] -> w673
                                tunnel: [w685] -> w677
                                tunnel: [w684] -> w676
                                tunnel: w675 -> [w686]
                                tunnel: w673 -> [w683]
                                frame #0 {
                                n222 = Wait (ms)(milliseconds to wait=u32 100) -> ()  [unwired: 1 out]
                                }
                                frame #1 {
                                n223 = VISA Write(VISA resource name=w683, write buffer="K", error in (no error)=w686) -> (VISA resource name out=w685:refnum<visa-resource-name>, error out=w684:errorcluster)  [unwired: 1 out]
                                }
                                }
                                }
                                frame 9, Default {
                                }
                                }
                              }
                              frame Disabled {
                                n224 = case shown="0, 기본" w691 {
                                frame 0, Default {
                                n225 = Current VI's Path() -> (path=w693:path)
                                n226 = Strip Path(path=w693) -> (stripped path=w694:path)  [unwired: 1 out]
                                n227 = Build Path(base path=w694, name or relative path="0.wav" ("이름 또는 상대 경로")) -> (appended path=w692:path)
                                n228 = call "Sound_Sub.vi"("path"=w692) -> ()
                                }
                                frame 2 {
                                n229 = Current VI's Path() -> (path=w696:path)
                                n230 = Strip Path(path=w696) -> (stripped path=w697:path)  [unwired: 1 out]
                                n231 = Build Path(base path=w697, name or relative path="2.wav" ("이름 또는 상대 경로")) -> (appended path=w699:path)
                                n232 = call "Sound_Sub.vi"("path"=w699) -> ()
                                }
                                frame 3 {
                                n233 = Current VI's Path() -> (path=w700:path)
                                n234 = Strip Path(path=w700) -> (stripped path=w701:path)  [unwired: 1 out]
                                n235 = Build Path(base path=w701, name or relative path="3.wav" ("이름 또는 상대 경로")) -> (appended path=w703:path)
                                n236 = call "Sound_Sub.vi"("path"=w703) -> ()
                                }
                                frame 4 {
                                n237 = Current VI's Path() -> (path=w704:path)
                                n238 = Strip Path(path=w704) -> (stripped path=w705:path)  [unwired: 1 out]
                                n239 = Build Path(base path=w705, name or relative path="4.wav" ("이름 또는 상대 경로")) -> (appended path=w707:path)
                                n240 = call "Sound_Sub.vi"("path"=w707) -> ()
                                }
                                frame 5 {
                                n241 = Current VI's Path() -> (path=w708:path)
                                n242 = Strip Path(path=w708) -> (stripped path=w709:path)  [unwired: 1 out]
                                n243 = Build Path(base path=w709, name or relative path="5.wav" ("이름 또는 상대 경로")) -> (appended path=w711:path)
                                n244 = call "Sound_Sub.vi"("path"=w711) -> ()
                                }
                                frame 1 {
                                n245 = Current VI's Path() -> (path=w713:path)
                                n246 = Strip Path(path=w713) -> (stripped path=w714:path)  [unwired: 1 out]
                                n247 = Build Path(base path=w714, name or relative path="1.wav" ("이름 또는 상대 경로")) -> (appended path=w712:path)
                                n248 = call "Sound_Sub.vi"("path"=w712) -> ()
                                }
                                }
                              }
                              frame Disabled {
                              }
                            }
                          }
                        }
                        n249 = global write "Control_Panel_정리.vi" "선택된 기능"(w577) -> ()
                      }
                      frame #1 {
                        n250 = global read "Control_Panel_정리.vi" "Send_Interaction"() -> (w717:u8)
                        n251 = stacked-sequence {
                          tunnel: w717 -> [w722 _ w727]
                          tunnel: u32 0 ("dwFlags") -> [w721 _ w726]
                          frame #0 {
                            n252 = dll-call lib="User32.dll" fn="keybd_event"("bVk"=w722, "bScan"=w721, "dwFlags"=w721, "dwExtraInfo"=w721) -> ()  [unwired: 8 in, 2 out]
                          }
                          frame #1 {
                            n253 = global write "Control_Panel_정리.vi" "Switch"(FALSE ("Switch")) -> ()
                            n254 = Wait Until Next ms Multiple(millisecond multiple=u32 250) -> ()  [unwired: 1 out]
                          }
                          frame #2 {
                            n255 = dll-call lib="User32.dll" fn="keybd_event"("bVk"=w727, "bScan"=w726, "dwFlags"=u32 2, "dwExtraInfo"=w726) -> ()  [unwired: 8 in, 2 out]
                          }
                        }
                      }
                    }
                  }
                  frame Disabled {
                    n256 = case shown="참" w729 {
                      tunnel: w730 -> [_ w733]
                      tunnel: ["No Decesion" ("메시지") w732] -> w728
                      frame False {
                      }
                      frame True {
                        n257 = disable-structure shown="활성화" {
                          disable-tunnel: [w735 _ "" ("메시지")] -> w732
                          disable-tunnel: w733 -> [w734 w743 _]
                          frame Enabled {
                            n258 = case shown="5" w734 {
                              tunnel: ["온도" ("메시지") "자판" ("메시지") "침대" ("메시지") "용변" ("메시지") "기계" ("메시지") "응급" ("메시지") "No Decesion" ("메시지")] -> w735
                              frame 0 {
                              }
                              frame 1 {
                              }
                              frame 2 {
                              }
                              frame 3 {
                              }
                              frame 4 {
                              }
                              frame 5 {
                              }
                              frame 9, Default {
                              }
                            }
                          }
                          frame Disabled {
                            n259 = case shown="4" w743 {
                              frame 0, Default {
                                n260 = Current VI's Path() -> (path=w745:path)
                                n261 = Strip Path(path=w745) -> (stripped path=w746:path)  [unwired: 1 out]
                                n262 = Build Path(base path=w746, name or relative path="0.wav" ("이름 또는 상대 경로")) -> (appended path=w744:path)
                                n263 = call "Sound_Sub.vi"("path"=w744) -> ()
                              }
                              frame 2 {
                                n264 = Current VI's Path() -> (path=w748:path)
                                n265 = Strip Path(path=w748) -> (stripped path=w749:path)  [unwired: 1 out]
                                n266 = Build Path(base path=w749, name or relative path="2.wav" ("이름 또는 상대 경로")) -> (appended path=w751:path)
                                n267 = call "Sound_Sub.vi"("path"=w751) -> ()
                              }
                              frame 3 {
                                n268 = Current VI's Path() -> (path=w752:path)
                                n269 = Strip Path(path=w752) -> (stripped path=w753:path)  [unwired: 1 out]
                                n270 = Build Path(base path=w753, name or relative path="3.wav" ("이름 또는 상대 경로")) -> (appended path=w755:path)
                                n271 = call "Sound_Sub.vi"("path"=w755) -> ()
                              }
                              frame 4 {
                                n272 = Current VI's Path() -> (path=w756:path)
                                n273 = Strip Path(path=w756) -> (stripped path=w757:path)  [unwired: 1 out]
                                n274 = Build Path(base path=w757, name or relative path="4.wav" ("이름 또는 상대 경로")) -> (appended path=w759:path)
                                n275 = call "Sound_Sub.vi"("path"=w759) -> ()
                              }
                              frame 5 {
                                n276 = Current VI's Path() -> (path=w760:path)
                                n277 = Strip Path(path=w760) -> (stripped path=w761:path)  [unwired: 1 out]
                                n278 = Build Path(base path=w761, name or relative path="5.wav" ("이름 또는 상대 경로")) -> (appended path=w763:path)
                                n279 = call "Sound_Sub.vi"("path"=w763) -> ()
                              }
                              frame 1 {
                                n280 = Current VI's Path() -> (path=w765:path)
                                n281 = Strip Path(path=w765) -> (stripped path=w766:path)  [unwired: 1 out]
                                n282 = Build Path(base path=w766, name or relative path="1.wav" ("이름 또는 상대 경로")) -> (appended path=w764:path)
                                n283 = call "Sound_Sub.vi"("path"=w764) -> ()
                              }
                            }
                          }
                          frame Disabled {
                          }
                        }
                      }
                    }
                    n284 = global write "Control_Panel_정리.vi" "선택된 기능"(w728) -> ()
                  }
                }
              }
            }
            n285 = Increment(x=w138) -> (x+1=w137:i32)
            n286 = Build Array (concatenate)(w147, w146) -> (w140:dbl[])
          }
        }
        n287 = global read "Control_Panel_정리.vi" "정지"() -> (w89:bool)
      }
      n288 = global write "Control_Panel_정리.vi" "Acquisition Mode"(TRUE ("Device Control Enabled")) -> ()
      n289 = global write "Control_Panel_정리.vi" "Device Control Enabled"(FALSE ("Device Control Enabled")) -> ()
    }
    frame #3 {
      n290 = VISA Close(VISA resource name=w771, error in (no error)=w770) -> ()  [unwired: 1 out]
      n291 = dll-call lib="C:/Users/Server/Desktop/NeuroSky/NeuroSky_Dll_Call/Debug/NeuroSky_Dll_Call.dll" fn="FreeConnection"() -> ()  [unwired: 4 in, 2 out]
      n292 = global write "Control_Panel_정리.vi" "Acquisition Mode"(FALSE ("Device Control Enabled")) -> ()
      n293 = global write "Control_Panel_정리.vi" "Communication Stopped"(TRUE ("Device Control Enabled")) -> ()
      n294 = Build Path(base path=w774, name or relative path="Brain.txt") -> (appended path=w813:path)
      n295 = Build Path(base path=w774, name or relative path="selectedtarget.txt") -> (appended path=w805:path)
      n296 = Build Path(base path=w774, name or relative path="mius_flash_order.txt") -> (appended path=w810:path)
      n297 = Build Path(base path=w774, name or relative path="Target_order.txt") -> (appended path=w800:path)
      n298 = Build Path(base path=w774, name or relative path="Accuracy.txt") -> (appended path=w803:path)
      n299 = Build Path(base path=w774, name or relative path="ERP_발생_total.txt") -> (appended path=w793:path)
      n300 = Build Path(base path=w774, name or relative path="ERP_all_icon.txt") -> (appended path=w789:path)
      n301 = Build Path(base path=w774, name or relative path="ERP_total.txt") -> (appended path=w777:path)
      n302 = Build Path(base path=w774, name or relative path="SWLDA_hyperplane_value.txt") -> (appended path=w785:path)
      n303 = Build Path(base path=w774, name or relative path="decision_value.txt") -> (appended path=w782:path)
      n304 = call-poly <vilib>:"Write To Spreadsheet File.vi"("format (%.3f)"="%.6f", "1D data"=w769, "file path (dialog if empty)"=w813) -> ()  [unwired: 5 in, 1 out]
      n305 = call-poly <vilib>:"Write To Spreadsheet File.vi"("1D data"=w804, "file path (dialog if empty)"=w805) -> ()  [unwired: 6 in, 1 out]
      n306 = call-poly <vilib>:"Write To Spreadsheet File.vi"("transpose? (no:F)"=TRUE, "2D data"=w808, "file path (dialog if empty)"=w810) -> ()  [unwired: 5 in, 1 out]
      n307 = call-poly <vilib>:"Write To Spreadsheet File.vi"("transpose? (no:F)"=TRUE, "1D data"=w797, "file path (dialog if empty)"=w800) -> ()  [unwired: 5 in, 1 out]
      n308 = call-poly <vilib>:"Write To Spreadsheet File.vi"("1D data"=w801, "file path (dialog if empty)"=w803) -> ()  [unwired: 6 in, 1 out]
      n309 = call-poly <vilib>:"Write To Spreadsheet File.vi"("transpose? (no:F)"=TRUE, "1D data"=w791, "file path (dialog if empty)"=w793) -> ()  [unwired: 5 in, 1 out]
      n310 = call-poly <vilib>:"Write To Spreadsheet File.vi"("transpose? (no:F)"=TRUE, "format (%.3f)"="%.6f", "2D data"=w786, "file path (dialog if empty)"=w789) -> ()  [unwired: 4 in, 1 out]
      n311 = call-poly <vilib>:"Write To Spreadsheet File.vi"("transpose? (no:F)"=TRUE, "format (%.3f)"="%.6f", "2D data"=w775, "file path (dialog if empty)"=w777) -> ()  [unwired: 4 in, 1 out]
      n312 = call-poly <vilib>:"Write To Spreadsheet File.vi"("format (%.3f)"="%.6f", "1D data"=w783, "file path (dialog if empty)"=w785) -> ()  [unwired: 5 in, 1 out]
      n313 = call-poly <vilib>:"Write To Spreadsheet File.vi"("format (%.3f)"="%.6f", "1D data"=w780, "file path (dialog if empty)"=w782) -> ()  [unwired: 5 in, 1 out]
    }
    frame #4 {
      n314 = global write "Control_Panel_정리.vi" "Communication Stopped"(FALSE ("Device Control Enabled")) -> ()
    }
  }
